vi "call complex and bools.vi"() -> ()   [LabVIEW 2022 SP3]
uses:
  <vilib>/Utility/error.llb/DialogType.ctl
panel:
  in  "Python version":string="3.9"
  out "String":string
  in  "function name":string="run"
  in  "module path":path=path "R:/work/LabVIEW-and-Python-interop/call complex and bools/call_complex_and_bools.py"
  in  "error in":errorcluster
  out "error out":errorcluster
  in  "Python path":path=path "C:/Users/Mikio Fukushima/AppData/Local/Programs/Python/Python39/python.exe"
  # "pythonスクリプトのパスに2バイトコードを含めるとエラーになるので注意。"
  # "Pythonノードを使用したLabVIEWへの/LabVIEWからのPythonデータ構造の受け渡し\nhttps://knowledge.ni.com/KnowledgeArticleDetails?id=kA03q000000oyaHCAQ&l=ja-JP"
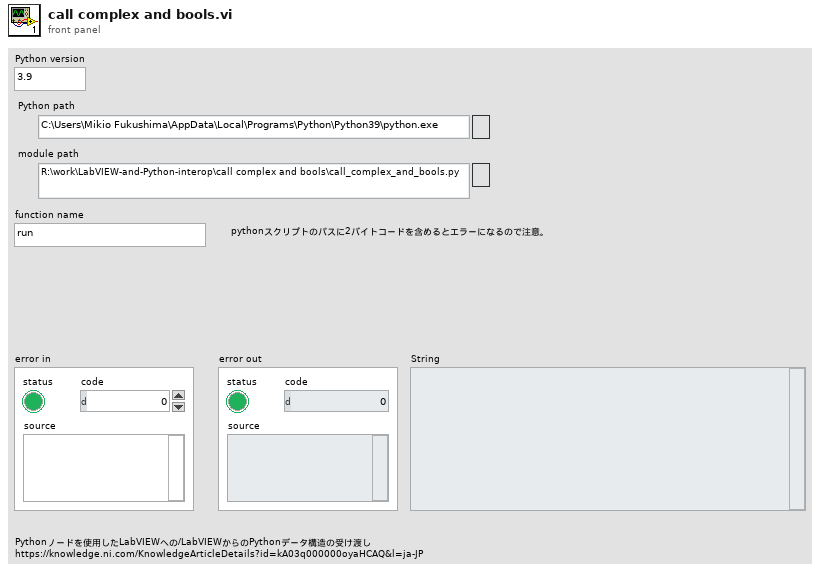
[diagram p1: front panel]
types:
  T1 = typedef "DialogType.ctl" = u16
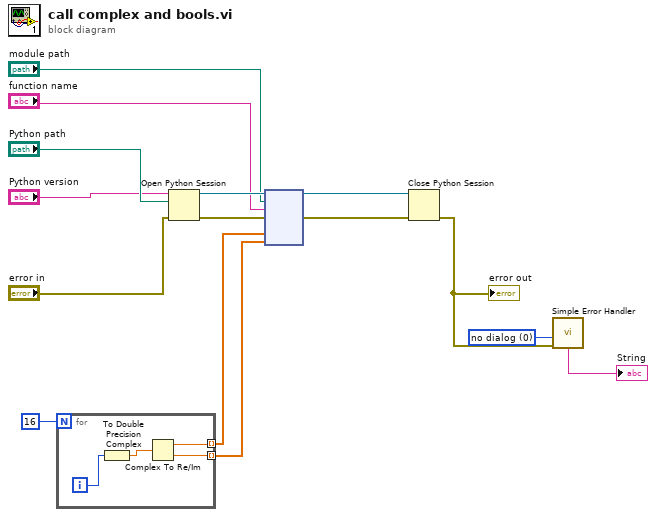
[diagram p0: block diagram]
diagram:
  w5 = T1 0 items=["no dialog", "OK message", "continue or stop message", "OK message + warnings", "continue/stop + warnings"] ("type of dialog (OK msg:1)")
  n1 = for {
    N: 16 -> [_]
    tunnel: [w18] -> w2 mode=indexing
    tunnel: [w17] -> w1 mode=indexing
    i -> [w19]
    n2 = To Double Precision Complex(1:w19) -> (0:w16:cdb)
    n3 = Complex To Re/Im(x + iy=w16) -> (x=w18:dbl, y=w17:dbl)
  }
  n4 = Open Python Session(python version="Python version", python path="Python path", 3:"error in") -> (session out=w13:refnum<k35>, error out=w10:errorcluster)
  n5 = node(w13, "module path", "function name", w10, w2, w1) -> (w12:refnum<k35>, w11:errorcluster)  [unwired: 4 in, 2 out]
  n6 = Close Python Session(session in=w12, error in=w11) -> (11:w7:errorcluster)
  "error out" <- w7
  n7 = call <vilib>:"Simple Error Handler.vi"("type of dialog (OK msg:1)"=w5, "error in (no error)"=w7) -> ("message"=→"String":string)  [unwired: 3 in, 4 out]
